vi "Unpack DBL.vi"(11 "Broadcast DBL Msg In":refnum<class "Broadcast DBL Msg.lvclass">) -> (2 "Value":dbl, 3 "Name":string)   [LabVIEW 2015, in "IViewable.lvlib" / "Broadcast DBL Msg.lvclass"]
uses:
  Broadcast DBL Msg.lvclass
  Broadcast DBL Msg.lvclass/Broadcast DBL Msg.ctl
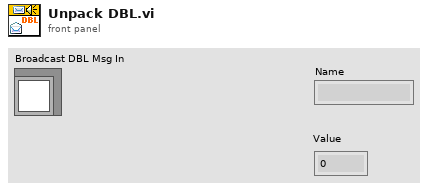
[diagram p1: front panel]
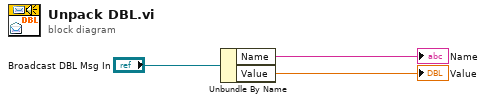
[diagram p0: block diagram]
diagram:
  n1 = Unbundle By Name("Broadcast DBL Msg In") -> ("Name"=→"Name":string, "Value"=→"Value":dbl)
